vi "Load Scaling Config.vi"(8 "error in (no error)":errorcluster, 11 "DataProcessor in":refnum<class "DataProcessor.lvclass">) -> (0 "error out":errorcluster, 3 "DataProcessor out":refnum<class "DataProcessor.lvclass">)   [LabVIEW 2020, in "Volatus.lvlib" / "DataProcessor.lvclass"]
uses:
  DataProcessor.lvclass
  C:/dev/lv20CE/relink/lv-volatus/Volatus/Task/Task.lvclass
  VolatusConfig/Scaling/Scaling.lvclass
  C:/dev/lv20CE/relink/lv-volatus/VolatusConfig/VolatusConfigElement/VolatusConfigElement.lvclass
  VolatusConfig/Meta Type.ctl
  VolatusConfig/SensorList/SensorList.lvclass
  DataProcessor.lvclass/DataProcessor.ctl
  VolatusConfig/VolatusConfigElement/VolatusConfigElement.lvclass/VolatusConfigElement.ctl
  VolatusConfig/Scale/Scale.lvclass
  lv-vecto/Vecto/Group/Group.lvclass
  C:/dev/lv20CE/relink/lv-vecto/Vecto/GroupAbstract/GroupAbstract.lvclass
  VolatusConfig/Task/Task.lvclass
  lv-cdm/CDM-Config/Config Lookup/Match Meta.vi
  lv-cdm/CDM-Config/Config Element/Owner.vi
  lv-cdm/CDM-Config/Config Manager/Lookup Descendant.vi
  lv-cdm/CDM-Config/Config Filter/Config Lookup.lvclass
  Task/Task.lvclass
  VolatusConfig/VolatusConfigElement/VolatusConfigElement.lvclass
  VolatusConfig/VolatusConfig.lvlib
  lv-cdm/CDM-Config/Config Element/Config Element.lvclass
  lv-vecto/Vecto/GroupAbstract/GroupAbstract.lvclass
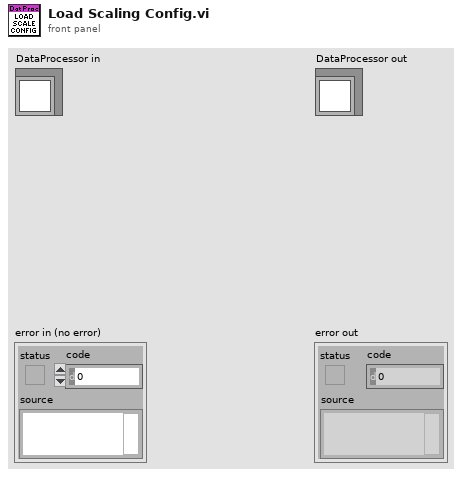
[diagram p1: front panel]
types:
  T1 = typedef "VolatusConfig.lvlib/Meta Type.ctl" = enum16{"UNKNOWN", "VL_System", "VL_Cluster", "VL_Node", "VL_Task", "VL_Group", "VL_Channel", "VL_Task_List", "VL_Scaling", "VL_Sensor", "VL_Sensor_List", "VL_Scale"}
  T2 = typedef "VolatusConfig.lvlib/Scale Type.ctl" = enum16{"None", "Sensor", "Polynomial", "Threshold"}
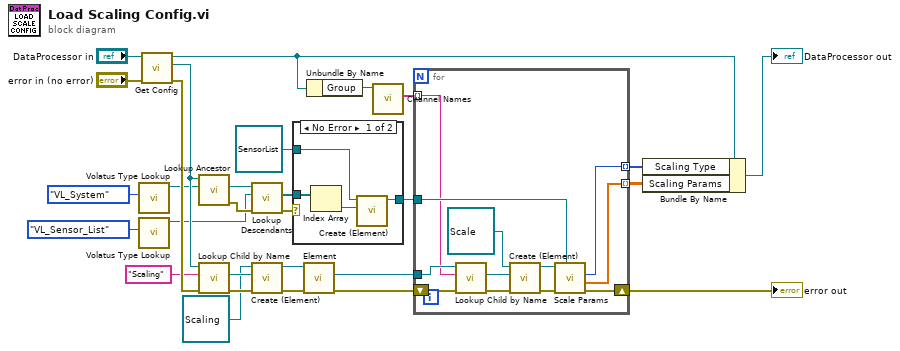
[diagram p0: block diagram]
diagram:
  n1 = call "Volatus Type Lookup.vi"("Meta Type"=Meta_Type."VL_System") -> ("Config Lookup out"=w19:refnum<class "Config Lookup.lvclass">)  [unwired: 9 in, 1 out]
  n2 = call "Volatus Type Lookup.vi"("Meta Type"=Meta_Type."VL_Sensor_List") -> ("Config Lookup out"=w15:refnum<class "Config Lookup.lvclass">)  [unwired: 9 in, 1 out]
  n3 = call "Get Config.vi"("error in (no error)"="error in (no error)", "Task in"="DataProcessor in") -> ("error out"=w27:errorcluster, "Config"=w20:refnum<class "Task.lvclass">, "Task out"=w3:refnum<class "DataProcessor.lvclass">)  [unwired: 7 in]
  n4 = call "Lookup Ancestor.vi"("Lookup"=w19, "VolatusConfigElement in"=w20) -> ("error out"=w26:errorcluster, "Ancestor"=w16:refnum<class "Config Element.lvclass">)  [unwired: 7 in, 1 out]
  n5 = call "Lookup Child by Name.vi"("error in (no error)"=w27, "Child Name"="Scaling", "VolatusConfigElement in"=w20) -> ("error out"=w28:errorcluster, "Child"=w22:refnum<class "Config Element.lvclass">)  [unwired: 5 in, 2 out]
  n6 = call "Lookup Descendants.vi"("error in (no error)"=w26, "Lookup"=w15, "Config Element in"=w16) -> ("error out"=w12:errorcluster, "Descendants"=w14:refnum<class "Config Element.lvclass">[])  [unwired: 6 in, 1 out]
  n7 = call "Create (Element).vi"("error in (no error)"=w28, "Element"=w22, "VolatusConfigElement in"=refnum<class "Scaling.lvclass"> refnum ("VolatusConfig.lvlib:Scaling.lvclass")) -> ("error out"=w9:errorcluster, "VolatusConfigElement out"=w11:refnum<class "Scaling.lvclass">)  [unwired: 7 in]
  n8 = case shown="No Error" w12 {
    tunnel: w14 -> [w32 _]
    tunnel: refnum<class "SensorList.lvclass"> refnum ("VolatusConfig.lvlib:SensorList.lvclass") -> [w30 _]
    tunnel: [w29 _] -> w10
    frame No Error {
      n9 = Index Array(array=w32) -> (element=w31:refnum<class "Config Element.lvclass">)  [unwired: 1 in]
      n10 = call "Create (Element).vi"("Element"=w31, "VolatusConfigElement in"=w30) -> ("VolatusConfigElement out"=w29:refnum<class "SensorList.lvclass">)  [unwired: 8 in, 1 out]
    }
    frame Error {
    }
  }
  n11 = call "Element.vi"("VolatusConfigElement in"=w11) -> ("Element"=w6:refnum<class "Config Element.lvclass">)  [unwired: 9 in, 1 out]
  n12 = Unbundle By Name(w3) -> ("Group"=w8:refnum<class "Group.lvclass">)
  n13 = call "Channel Names.vi"("GroupAbstract in"=w8) -> ("Channel Names"=w7:string[])  [unwired: 8 in, 2 out]
  n14 = for {
    tunnel: w10 -> [w41]
    shift-right: [w33] -> w1
    shift-left: w9 -> [w40]
    tunnel: w7 -> [w38] mode=indexing
    tunnel: w6 -> [w39]
    tunnel: [w35] -> w5 mode=indexing
    tunnel: [w34] -> w4 mode=indexing
    n15 = call "Lookup Child by Name.vi"("error in (no error)"=w40, "Name"=w38, "Config Element in"=w39) -> ("error out"=w36:errorcluster, "Child"=w37:refnum<class "Config Element.lvclass">)  [unwired: 5 in, 2 out]
    n16 = call "Create (Element).vi"("error in (no error)"=w36, "Element"=w37, "VolatusConfigElement in"=refnum<class "Scale.lvclass"> refnum ("VolatusConfig.lvlib:Scale.lvclass")) -> ("error out"=w42:errorcluster, "VolatusConfigElement out"=w43:refnum<class "Scale.lvclass">)  [unwired: 7 in]
    n17 = call "Scale Params.vi"("SensorList (Auto)"=w41, "error in (no error)"=w42, "Scale in"=w43) -> ("error out"=w33:errorcluster, "Scale Params"=w34:dbl[], "Scale Type"=w35:T2)  [unwired: 5 in, 1 out]
  }
  "error out" <- w1
  n18 = Bundle By Name(cluster=w3, "Scaling Type"=w5, "Scaling Params"=w4) -> (→"DataProcessor out":refnum<class "DataProcessor.lvclass">)
